vi "transmit.vi"(8 "error in (no error)":errorcluster, 10 "RESP3 Value":variant, 11 "Test Redis Client in":refnum<class "Test Redis Client.lvclass">) -> (0 "error out":errorcluster, 3 "Test Redis Client out":refnum<class "Test Redis Client.lvclass">)   [LabVIEW 2019, in "Test Redis Client for LabVIEW.lvlib" / "Test Redis Client.lvclass"]
uses:
  Test Redis Client.lvclass
  RESP3 for LabVIEW/RESP3/RESP3.lvlib
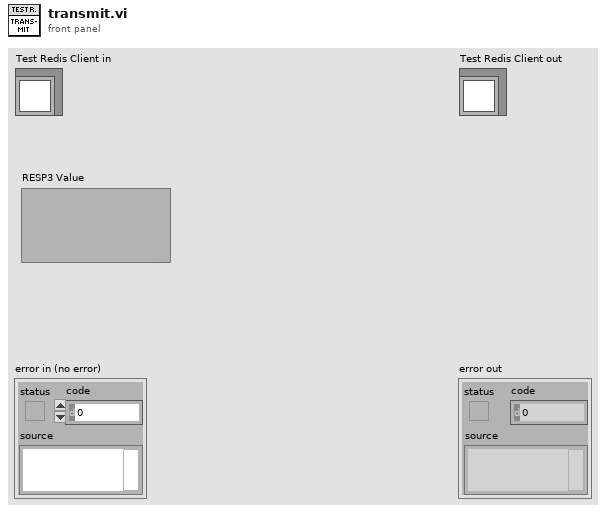
[diagram p1: front panel]
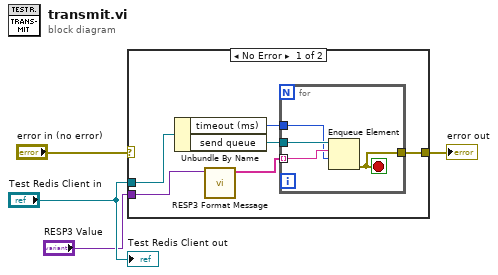
[diagram p0: block diagram]
diagram:
  n1 = case shown="No Error" "error in (no error)" {
    selector: "error in (no error)" -> [_ w15]
    tunnel: "Test Redis Client in" -> [w10 _]
    tunnel: [w8 w15] -> w2
    tunnel: "RESP3 Value" -> [w6 _]
    frame No Error {
      n2 = Unbundle By Name(w10) -> ("timeout (ms)"=w7:i32, "send queue"=w9:refnum<queue>)
      n3 = call "RESP3 Format Message.vi"("RESP3 Value"=w6) -> ("messages"=w5:string[])  [unwired: 9 in, 1 out]
      n4 = for {
        tunnel: w9 -> [w14]
        tunnel: w5 -> [w13] mode=indexing
        tunnel: [w12] -> w8
        tunnel: w7 -> [w11]
        stop <- w12 stop-if-true
        n5 = Enqueue Element(queue=w14, element=w13, timeout in ms (-1)=w11) -> (error out=w12:errorcluster)  [unwired: 1 in, 2 out]
      }
    }
    frame Error {
    }
  }
  "error out" <- w2
  "Test Redis Client out" <- "Test Redis Client in"
